vi "Experiment RT Servo.vi"(10 "Experiment Inputs":T2={"Duration"=5.0, "Initialisation Time"=1.0, "Sample Rate (Hz)"=200.0, "signal_type"=enum."Square", "Frequency"=0.5, "Amplitude"=1.0, "Offset"=2.5, "Velocity_feedback_gain"=0.1, "Feedforward_gain"=0.8, "LED_GAIN"=0.0, "LED_OFFSET"=0.0, "initial_condition"=0.0}) -> (0 "Error Out":errorcluster)   [LabVIEW 2016]
uses:
  Controls/Experiment Inputs.ctl
  Controls/Signal Type.ctl
  RT - Controls/Experiment RT State.ctl
  RT - Controls/Machine Data - RT.ctl
  <vilib>/Platform/TimedLoop/XDataNode/timing_clust.ctl
  <vilib>/Platform/TimedLoop/XDataNode/nitl_modes.ctl
  <vilib>/Platform/TimedLoop/XDataNode/wakeup.ctl
  Controller/Controller Values.ctl
  Controls/Experiment Outputs.ctl
  Pauseable Timer/Timer Mode.ctl
  <vilib>/Platform/TimedLoop/XDataNode/XDataNode.xnode
  <vilib>/ptbypt/NI_PtbyPt.lvlib
  <vilib>/Platform/TimedLoop/XDataNode/XDNodeRunTimeDep.lvlib
panel:
  out "Experiment RT State":T1
  in  "Error In":errorcluster
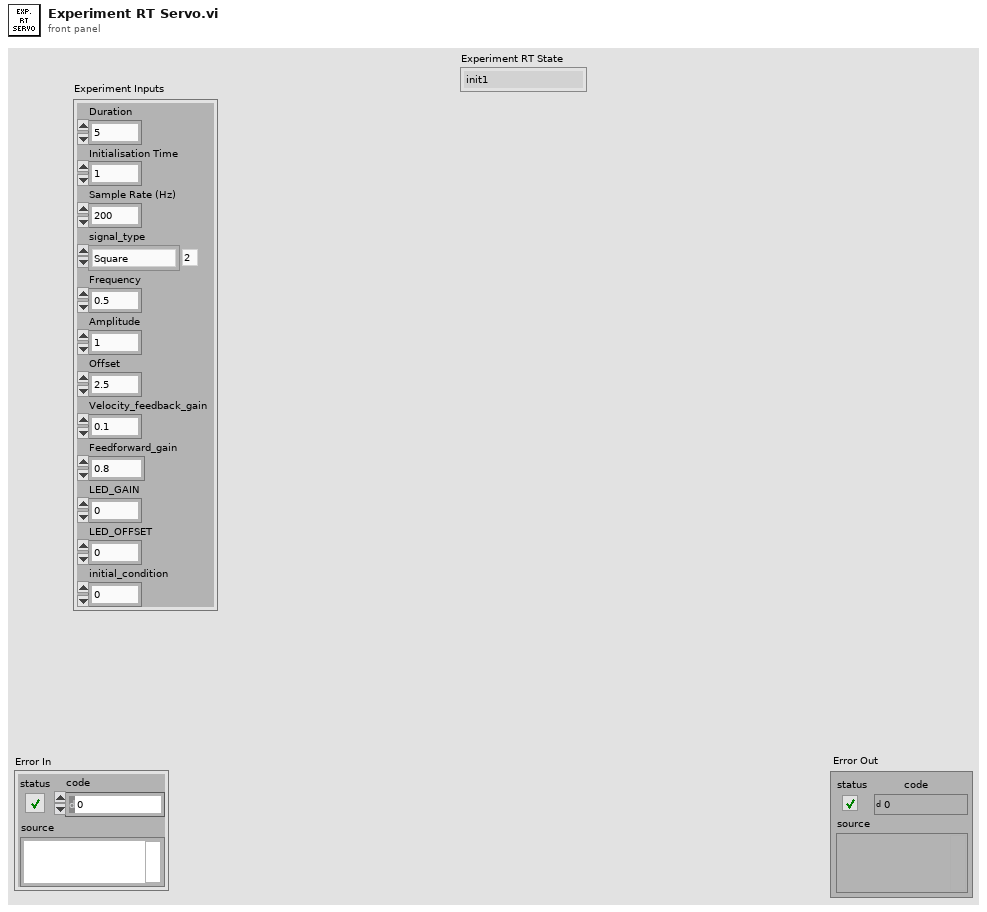
[diagram p1: front panel]
types:
  T1 = typedef "Experiment RT State.ctl" = enum16{"init1", "wait", "setup", "Initialise", "Wait Initialise", "Experiment", "End Experiment", "publisharray1", "publisharray2", "publisharray3", "publishspreadsheet"}
  T2 = typedef "Experiment Inputs.ctl" = cluster{"Duration":dbl, "Initialisation Time":dbl, "Sample Rate (Hz)":dbl, "signal_type":T3, "Frequency":dbl, "Amplitude":dbl, "Offset":dbl, "Velocity_feedback_gain":dbl, "Feedforward_gain":dbl, "LED_GAIN":dbl, "LED_OFFSET":dbl, "initial_condition":dbl}
  T3 = typedef "Signal Type.ctl" = enum16{"Sine", "Cosine", "Square", "Step"}
  T4 = typedef "Machine Data - RT.ctl" = cluster{"Results Array":dbl[][], "Motor Output":dbl, "LED Output":dbl, "Sample Index":u32, "Req. Samples":u32}
  T5 = typedef "XDNodeRunTimeDep.lvlib/timing_clust.ctl" = cluster{"Expected End [f-1]":u64, "Actual End [f-1]":u64, "Finished Late? [f-1]":bool, "Expected End [i-1]":u64, "Actual End [i-1]":u64, "Finished Late? [i-1]":bool, "Expected Start [i]":u64, "Actual Start [i]":u64, "Expected Start [f]":u64, "Actual Start [f]":u64, "Source Name":string, "Structure Name":string, "Period":i64, "Deadline":i64, "Offset":i64, "Start":i64, "Priority":i32, "Timeout":i32, "Mode":T6, "Wakeup Reason":T7, "Error":errorcluster, "Source Type":string, "Secondary Source Type":string, "Global End Time":u64, "Global Start Time":u64, "Frame Duration":u64, "Iteration Duration":u64, "Assigned CPU":i32, "I/O Scan Engine Mode":u32}
  T6 = typedef "XDNodeRunTimeDep.lvlib/nitl_modes.ctl" = enum32{"No Change", "Process missed periods, maintain original phase", "Discard missed periods, maintain original phase", "Process missed periods, ignore original phase", "Discard missed periods, ignore original phase"}
  T7 = typedef "XDNodeRunTimeDep.lvlib/wakeup.ctl" = enum32{"Normal", "Aborted", "Asynchronous wakeup", "Timing source error", "Timed loop error", "Timeout"}
  T8 = typedef "Controller Values.ctl" = cluster{"Ka":dbl, "Kt":dbl, "Offset":dbl}
  T9 = typedef "Timer Mode.ctl" = enum16{"Initialise", "Read", "Pause"}
  T10 = typedef "Experiment Outputs.ctl" = cluster{"Results Array":dbl[][], "spreadsheet":string}
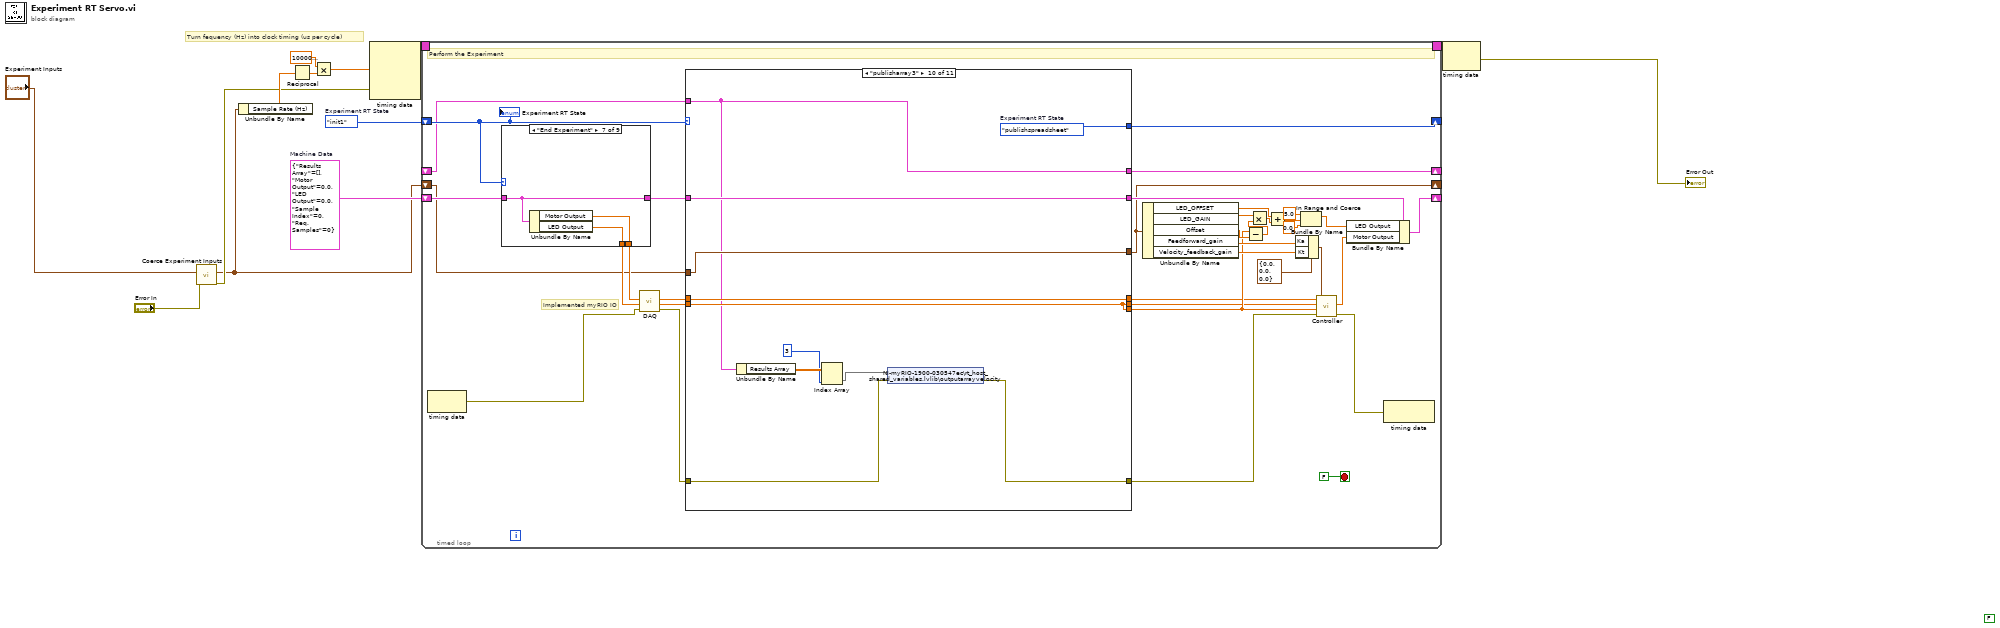
[diagram p0: block diagram]
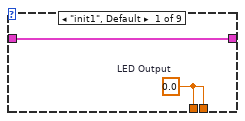
[diagram p2: hidden frame]
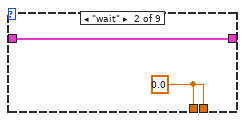
[diagram p3: hidden frame]
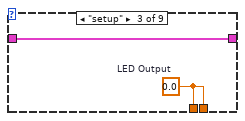
[diagram p4: hidden frame]
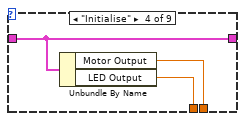
[diagram p5: hidden frame]
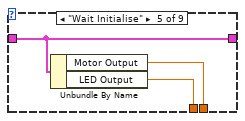
[diagram p6: hidden frame]
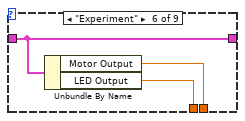
[diagram p7: hidden frame]
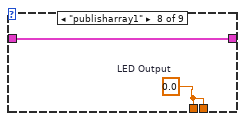
[diagram p8: hidden frame]
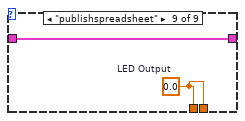
[diagram p9: hidden frame]
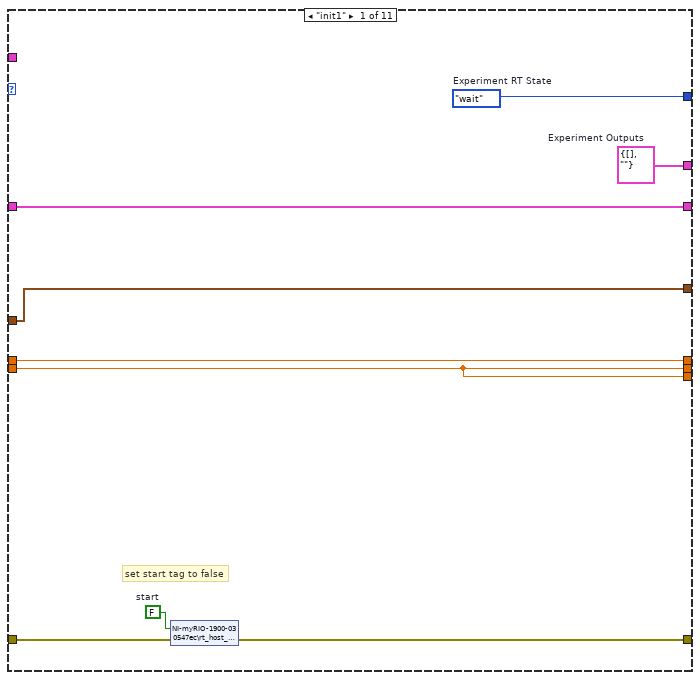
[diagram p10: hidden frame]
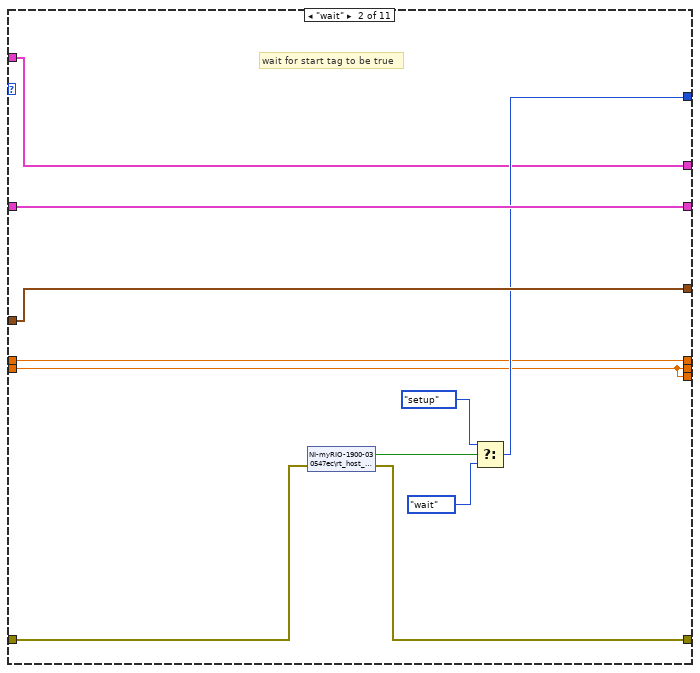
[diagram p11: hidden frame]
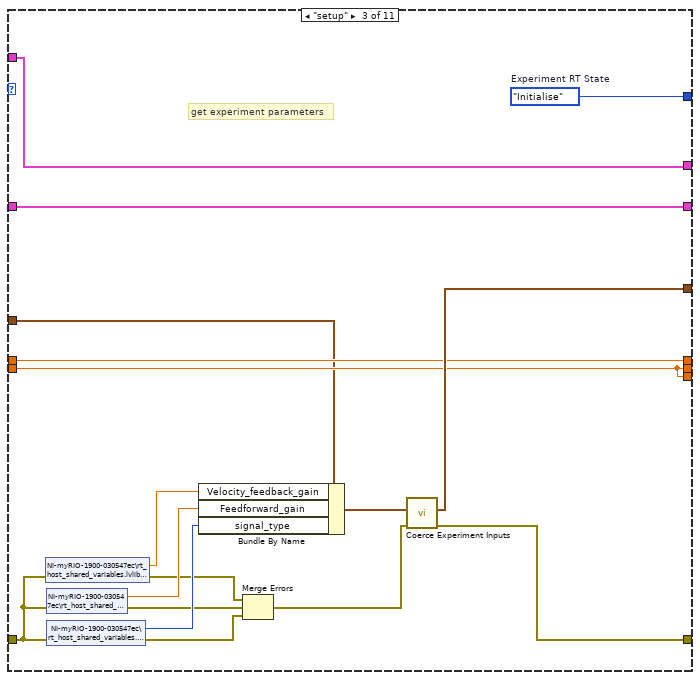
[diagram p12: hidden frame]
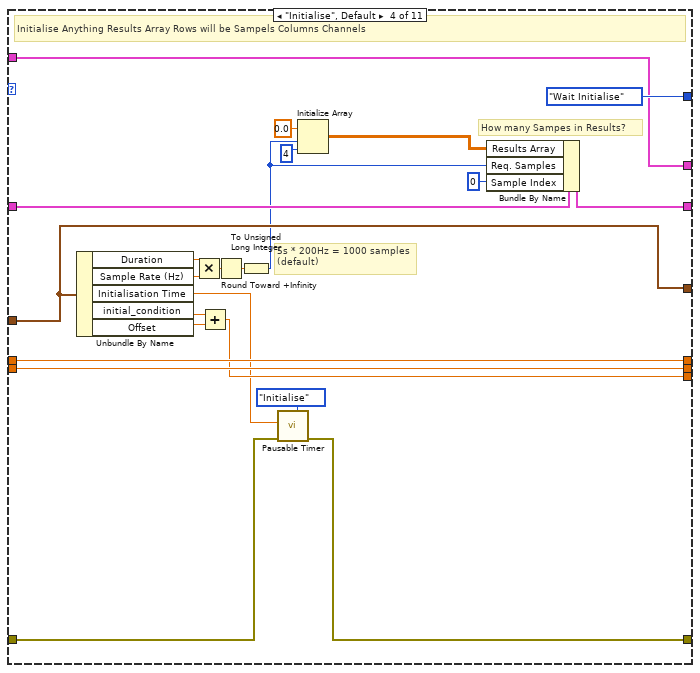
[diagram p13: hidden frame]
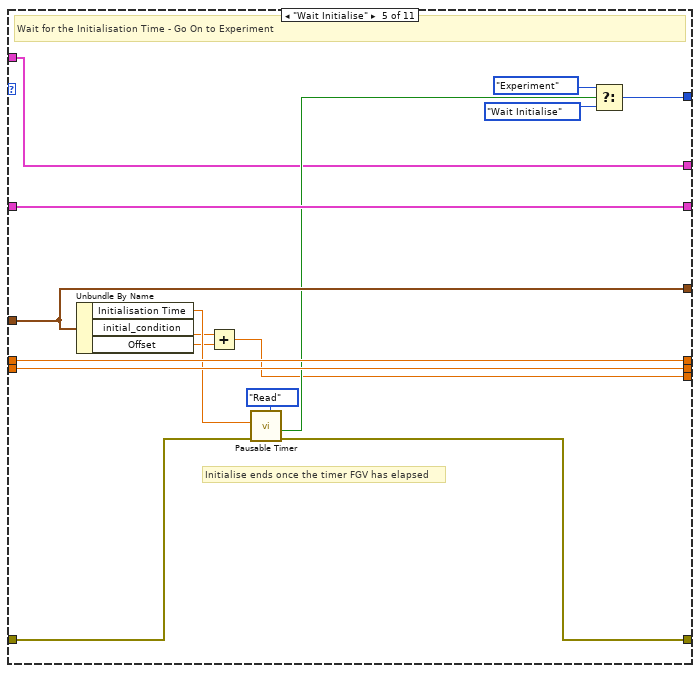
[diagram p14: hidden frame]
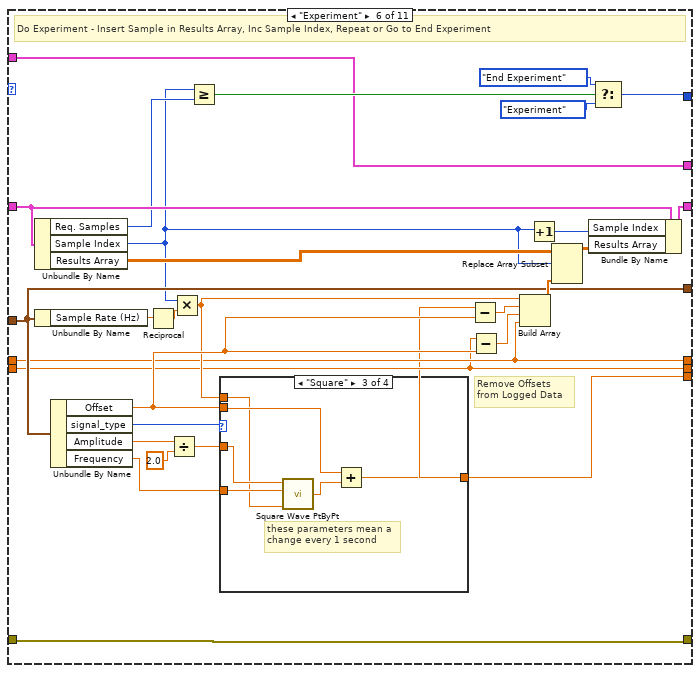
[diagram p15: hidden frame]
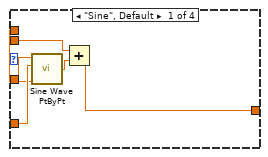
[diagram p16: hidden frame]
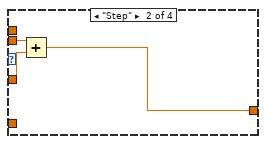
[diagram p17: hidden frame]
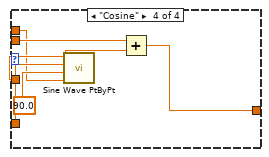
[diagram p18: hidden frame]
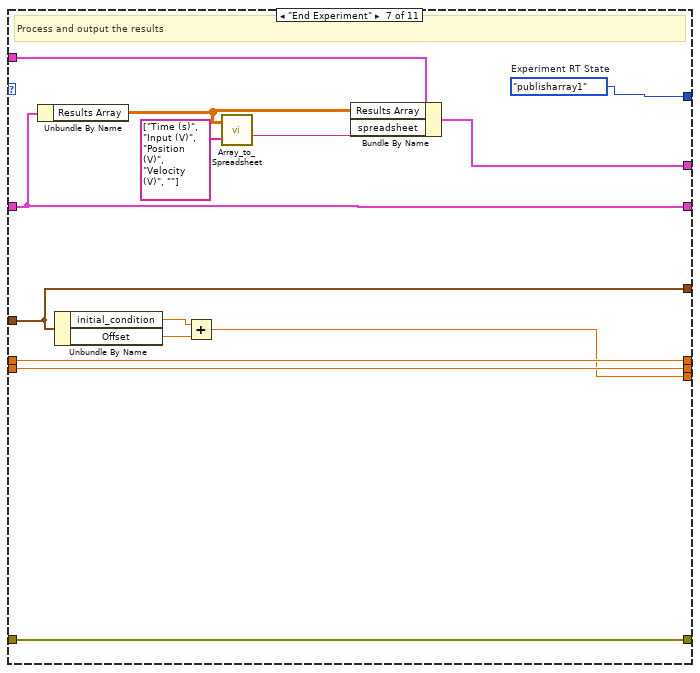
[diagram p19: hidden frame]
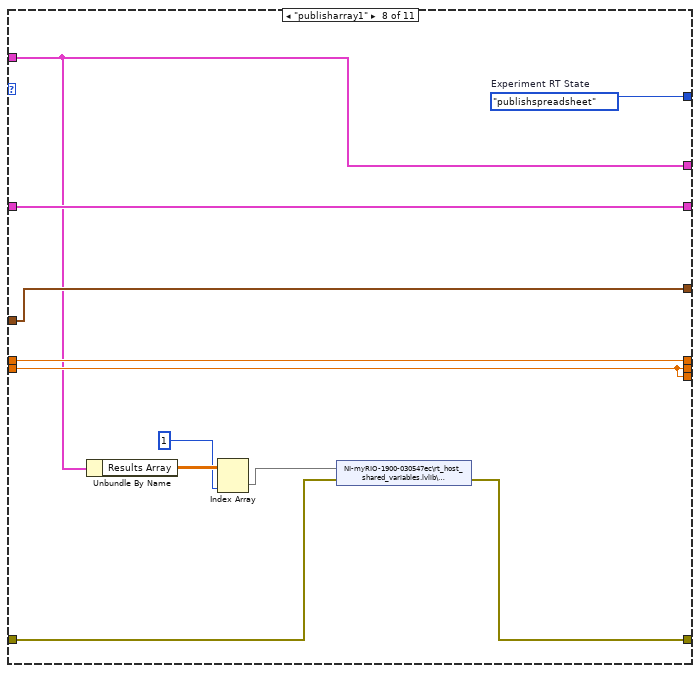
[diagram p20: hidden frame]
diagram:
  (unwired) FALSE
  w5 = T4 {"Results Array"=[], "Motor Output"=0.0, "LED Output"=0.0, "Sample Index"=0, "Req. Samples"=0}  # Machine Data
  w11 = Experiment_RT_State."init1"  # Experiment RT State
  # "Turn fequency (Hz) into clock timing (us per cycle)"
  n1 = call "Coerce Experiment Inputs.vi"("Error In"="Error In", "Experiment Inputs"="Experiment Inputs") -> ("Error Out"=w6:errorcluster, "Experiment Inputs Out"=w1:T2)  [unwired: 8 in]
  n2 = Unbundle By Name(w1) -> ("Sample Rate (Hz)"=w10:dbl)
  n3 = Reciprocal(x=w10) -> (1/x=w9:dbl)
  n4 = Multiply(x=1000000.0 ("y"), y=w9) -> (x*y=w7:dbl)
  n5 = node-c288(w7, w6) -> (w13:T5)  [unwired: 2 in]
  n6 = timed-loop {
    shift-right: [w45] -> _
    shift-left: w11 -> [w17]
    shift-right: [w48] -> _
    shift-left: w5 -> [w49]
    timing: w13 -> [_]
    timing-out: [_] -> w12
    shift-right: [w32] -> _
    shift-left: w1 -> [w18]
    shift-right: [w44] -> _
    shift-left: _ -> [w15]
    stop <- FALSE stop-if-true
    # "Implemented myRIO IO"
    # "Perform the Experiment"
    n7 = node-c288() -> (w46:errorcluster)  [unwired: 1 in]
    n8 = case shown="\"End Experiment\"" w17 {
      tunnel: w49 -> [w51 w53 w55 w58 w61 w64 w67 w69 w71]
      tunnel: [w50 w52 w54 w57 w60 w63 w66 w68 w70] -> w36
      tunnel: [w50 w52 w54 w56 w59 w62 w65 w68 w70] -> w22
      tunnel: [w51 w53 w55 w58 w61 w64 w67 w69 w71] -> w16
      frame "init1", Default {
        w50 = 0.0  # LED Output
      }
      frame "wait" {
        w52 = 0.0
      }
      frame "setup" {
        w54 = 0.0  # LED Output
      }
      frame "Initialise" {
        n9 = Unbundle By Name(w58) -> ("Motor Output"=w56:dbl, "LED Output"=w57:dbl)
      }
      frame "Wait Initialise" {
        n10 = Unbundle By Name(w61) -> ("Motor Output"=w59:dbl, "LED Output"=w60:dbl)
      }
      frame "Experiment" {
        n11 = Unbundle By Name(w64) -> ("Motor Output"=w62:dbl, "LED Output"=w63:dbl)
      }
      frame "End Experiment" {
        n12 = Unbundle By Name(w67) -> ("Motor Output"=w65:dbl, "LED Output"=w66:dbl)
      }
      frame "publisharray1" {
        w68 = 0.0  # LED Output
      }
      frame "publishspreadsheet" {
        w70 = 0.0  # LED Output
      }
    }
    n13 = call "DAQ.vi"("Error In"=w46, "LED Output"=w36, "Motor Output"=w22) -> ("Error Out"=w38:errorcluster, "Position FB"=w23:dbl, "Tacho FB"=w24:dbl)  [unwired: 4 in, 2 out]
    n14 = case shown="\"publisharray3\"" w17 {
      tunnel: [w72 w88 w107 w129 w147 w161 w200 w214 w226 w236 w249] -> w43
      tunnel: w18 -> [w78 w91 w101 w125 w146 w165 w210 w221 w232 w243 w252]
      tunnel: w16 -> [w75 w90 w103 w131 w142 w176 w209 w222 w233 w244 w253]
      tunnel: [w75 w90 w103 w130 w142 w175 w209 w222 w233 w244 w253] -> w37
      tunnel: [w78 w91 w106 w125 w146 w165 w210 w221 w232 w243 w252] -> w32
      tunnel: w38 -> [w79 w89 w102 w123 w145 w161 w200 w213 w225 w235 w250]
      tunnel: [w76 w82 w104 w124 w134 w149 w204 w219 w230 w241 w251] -> w25
      tunnel: w24 -> [w77 w83 w105 w128 w144 w156 w212 w220 w231 w242 w251]
      tunnel: [w77 w83 w105 w128 w144 w156 w212 w220 w231 w242 w251] -> w20
      tunnel: [w76 w82 w104 w127 w143 w155 w211 w219 w230 w241 w251] -> w19
      tunnel: w23 -> [w76 w82 w104 w127 w143 w155 w211 w219 w230 w241 _]
      tunnel: [w73 w84 w108 Experiment_RT_State."Wait Initialise" ("Experiment RT State") w141 w173 w199 w223 w234 w245 w254] -> w45
      tunnel: [w74 w81 w92 w109 w132 w148 w202 w218 w229 w240 w247] -> w44
      tunnel: w15 -> [_ w81 w92 w109 w132 w148 w201 w218 w229 w240 w247]
      frame "init1" {
        w73 = Experiment_RT_State."wait"  # Experiment RT State
        w74 = T10 {"Results Array"=[], "spreadsheet"=""}  # Experiment Outputs
        w80 = FALSE  # start
        # "set start tag to false"
        n15 = shared-variable "NI-myRIO-1900-030547ec\\rt_host_shared_variables.lvlib\\start"(w80, error in=w79) -> (error out=w72:errorcluster)
      }
      frame "wait" {
        # "wait for start tag to be true"
        n16 = shared-variable "NI-myRIO-1900-030547ec\\rt_host_shared_variables.lvlib\\start"(error in=w89) -> (w87:bool, error out=w88:errorcluster)
        n17 = Select(t=Experiment_RT_State."setup" ("Experiment RT State"), s=w87, f=Experiment_RT_State."wait" ("Experiment RT State")) -> (s? t:f=w84:T1)
      }
      frame "setup" {
        w108 = Experiment_RT_State."Initialise"  # Experiment RT State
        # "get experiment parameters"
        n18 = shared-variable "NI-myRIO-1900-030547ec\\rt_host_shared_variables.lvlib\\vel_fb_gain"(error in=w102) -> (w100:dbl, error out=w96:errorcluster)
        n19 = shared-variable "NI-myRIO-1900-030547ec\\rt_host_shared_variables.lvlib\\ff_gain"(error in=w102) -> (w99:dbl, error out=w95:errorcluster)
        n20 = shared-variable "NI-myRIO-1900-030547ec\\rt_host_shared_variables.lvlib\\signaltype"(error in=w102) -> (w98:u32, error out=w94:errorcluster)
        n21 = Bundle By Name(cluster=w101, "Velocity_feedback_gain"=w100, "Feedforward_gain"=w99, "signal_type"=w98) -> (w97:T2)
        n22 = Merge Errors(w96, w95, w94) -> (w93:errorcluster)
        n23 = call "Coerce Experiment Inputs.vi"("Error In"=w93, "Experiment Inputs"=w97) -> ("Error Out"=w107:errorcluster, "Experiment Inputs Out"=w106:T2)  [unwired: 8 in]
      }
      frame "Initialise", Default {
        # "5s * 200Hz = 1000 samples\n(default)"
        # "How many Sampes in Results?"
        # "Initialise Anything Results Array Rows will be Sampels Columns Channels"
        n24 = Unbundle By Name(w125) -> ("Duration"=w121:dbl, "Sample Rate (Hz)"=w120:dbl, "Initialisation Time"=w122:dbl, "initial_condition"=w112:dbl, "Offset"=w111:dbl)
        n25 = Multiply(x=w121, y=w120) -> (x*y=w119:dbl)
        n26 = Add(x=w112, y=w111) -> (x+y=w124:dbl)
        n27 = Round Toward +Infinity(x=w119) -> (ceil(x): smallest int >= x=w118:dbl)
        n28 = To Unsigned Long Integer(number=w118) -> (unsigned 32bit integer=w113:u32)
        n29 = call "Pausable Timer.vi"("Timer Mode"=Timer_Mode."Initialise", "Error In"=w123, "Desired Time (S)"=w122) -> ("Error Out"=w129:errorcluster)  [unwired: 6 in, 2 out]
        n30 = Initialize Array(0.0 ("element"), w113, 4 ("dimension size")) -> (w115:dbl[][])
        n31 = Bundle By Name(cluster=w131, "Results Array"=w115, "Req. Samples"=w113, "Sample Index"=u32 0) -> (w130:T4)
      }
      frame "Wait Initialise" {
        # "Initialise ends once the timer FGV has elapsed"
        # "Wait for the Initialisation Time - Go On to Experiment"
        n32 = Unbundle By Name(w146) -> ("Initialisation Time"=w140:dbl, "initial_condition"=w135:dbl, "Offset"=w133:dbl)
        n33 = Add(x=w135, y=w133) -> (x+y=w134:dbl)
        n34 = call "Pausable Timer.vi"("Timer Mode"=Timer_Mode."Read", "Error In"=w145, "Desired Time (S)"=w140) -> ("Error Out"=w147:errorcluster, "Time Up?"=w139:bool)  [unwired: 6 in, 1 out]
        n35 = Select(t=Experiment_RT_State."Experiment" ("Experiment RT State"), s=w139, f=Experiment_RT_State."Wait Initialise" ("Experiment RT State")) -> (s? t:f=w141:T1)
      }
      frame "Experiment" {
        # "Remove Offsets\nfrom Logged Data"
        # "Do Experiment - Insert Sample in Results Array, Inc Sample Index, Repeat or Go to End Experiment"
        n36 = Unbundle By Name(w176) -> ("Req. Samples"=w169:u32, "Sample Index"=w164:u32, "Results Array"=w167:dbl[][])
        n37 = Unbundle By Name(w165) -> ("Sample Rate (Hz)"=w163:dbl)
        n38 = Unbundle By Name(w165) -> ("Offset"=w158:dbl, "signal_type"=w160:T3, "Amplitude"=w151:dbl, "Frequency"=w159:dbl)
        n39 = Reciprocal(x=w163) -> (1/x=w162:dbl)
        n40 = Divide(x=w151, y=2.0) -> (x/y=w152:dbl)
        n41 = Multiply(x=w164, y=w162) -> (x*y=w157:dbl)
        n42 = Greater Or Equal?(x=w164, y=w169) -> (x >= y?=w170:bool)
        n43 = case shown="\"Square\"" w160 {
          tunnel: w152 -> [w182 w184 w191 w197]
          tunnel: w159 -> [w181 _ w190 w196]
          tunnel: w158 -> [w179 w185 w188 w193]
          tunnel: [w178 w183 w186 w194] -> w149
          tunnel: w157 -> [w177 _ w187 w192]
          frame "Sine", Default {
            n44 = call <vilib>:"Sine Wave PtByPt.vi"("time"=w177, "frequency"=w181, "amplitude"=w182) -> ("sine wave"=w180:dbl)  [unwired: 1 in]
            n45 = Add(x=w179, y=w180) -> (x+y=w178:dbl)
          }
          frame "Step" {
            n46 = Add(x=w185, y=w184) -> (x+y=w183:dbl)
          }
          frame "Square" {
            # "these parameters mean a\nchange every 1 second"
            n47 = call <vilib>:"Square Wave PtByPt.vi"("amplitude"=w191, "frequency"=w190, "time"=w187) -> ("square wave"=w189:dbl)  [unwired: 2 in]
            n48 = Add(x=w188, y=w189) -> (x+y=w186:dbl)
          }
          frame "Cosine" {
            n49 = call <vilib>:"Sine Wave PtByPt.vi"("time"=w192, "phase"=90.0, "frequency"=w196, "amplitude"=w197) -> ("sine wave"=w195:dbl)
            n50 = Add(x=w193, y=w195) -> (x+y=w194:dbl)
          }
        }
        n51 = Subtract(x=w149, y=w158) -> (x-y=w154:dbl)
        n52 = Subtract(x=w155, y=w158) -> (x-y=w153:dbl)
        n53 = Build Array(w157, w154, w153, w156) -> (w166:dbl[])
        n54 = Increment(x=w164) -> (x+1=w174:u32)
        n55 = Replace Array Subset(array=w167, new element=w166, index (row)=w164) -> (w168:dbl[][])  [unwired: 1 in]
        n56 = Bundle By Name(cluster=w176, "Sample Index"=w174, "Results Array"=w168) -> (w175:T4)
        n57 = Select(t=Experiment_RT_State."End Experiment" ("Experiment RT State"), s=w170, f=Experiment_RT_State."Experiment" ("Experiment RT State")) -> (s? t:f=w173:T1)
      }
      frame "End Experiment" {
        w199 = Experiment_RT_State."publisharray1"  # Experiment RT State
        # "Process and output the results"
        n58 = Unbundle By Name(w209) -> ("Results Array"=w203:dbl[][])
        n59 = Unbundle By Name(w210) -> ("initial_condition"=w205:dbl, "Offset"=w206:dbl)
        n60 = Add(x=w205, y=w206) -> (x+y=w204:dbl)
        n61 = call "Array_to_Spreadsheet.vi"("Headers"=string[] ["Time (s)", "Input (V)", "Position (V)", "Velocity (V)", ""], "Input Array"=w203) -> ("spreadsheet string"=w208:string)
        n62 = Bundle By Name(cluster=w201, "Results Array"=w203, "spreadsheet"=w208) -> (w202:T10)
      }
      frame "publisharray1" {
        w223 = Experiment_RT_State."publishspreadsheet"  # Experiment RT State
        n63 = Unbundle By Name(w218) -> ("Results Array"=w217:dbl[][])
        n64 = Index Array(array=w217, index (col)=1 ("disabled index (col)")) -> (element=w215:dbl[])  [unwired: 1 in]
        n65 = shared-variable "NI-myRIO-1900-030547ec\\rt_host_shared_variables.lvlib\\outputarrayinput"(w215, error in=w213) -> (error out=w214:errorcluster)
      }
      frame "publisharray2" {
        w234 = Experiment_RT_State."publishspreadsheet"  # Experiment RT State
        n66 = Unbundle By Name(w229) -> ("Results Array"=w228:dbl[][])
        n67 = Index Array(array=w228, index (col)=2 ("disabled index (col)")) -> (element=w224:dbl[])  [unwired: 1 in]
        n68 = shared-variable "NI-myRIO-1900-030547ec\\rt_host_shared_variables.lvlib\\outputarrayposition"(w224, error in=w225) -> (error out=w226:errorcluster)
      }
      frame "publisharray3" {
        w245 = Experiment_RT_State."publishspreadsheet"  # Experiment RT State
        n69 = Unbundle By Name(w240) -> ("Results Array"=w239:dbl[][])
        n70 = Index Array(array=w239, index (col)=3 ("disabled index (col)")) -> (element=w237:dbl[])  [unwired: 1 in]
        n71 = shared-variable "NI-myRIO-1900-030547ec\\rt_host_shared_variables.lvlib\\outputarrayvelocity"(w237, error in=w235) -> (error out=w236:errorcluster)
      }
      frame "publishspreadsheet" {
        w254 = Experiment_RT_State."init1"  # Experiment RT State
        n72 = Unbundle By Name(w247) -> ("spreadsheet"=w246:string)
        n73 = To Variant(anything=w246) -> (Variant=w248:variant)
        n74 = shared-variable "NI-myRIO-1900-030547ec\\rt_host_shared_variables.lvlib\\Output"(w248, error in=w250) -> (error out=w249:errorcluster)
      }
    }
    n75 = Unbundle By Name(w32) -> ("LED_OFFSET"=w33:dbl, "LED_GAIN"=w35:dbl, "Offset"=w30:dbl, "Feedforward_gain"=w40:dbl, "Velocity_feedback_gain"=w39:dbl)
    n76 = Subtract(x=w25, y=w30) -> (x-y=w31:dbl)
    n77 = Multiply(x=w35, y=w31) -> (x*y=w34:dbl)
    n78 = Add(x=w33, y=w34) -> (x+y=w29:dbl)
    n79 = Bundle By Name(cluster=T8 {"Ka"=0.0, "Kt"=0.0, "Offset"=0.0} ("Controller Values"), "Ka"=w40, "Kt"=w39) -> (w41:T8)
    n80 = In Range and Coerce(upper limit=5.0, x=w29, lower limit=0.0) -> (coerced(x)=w26:dbl)  [unwired: 1 out]
    n81 = call "Controller.vi"("Controller Values"=w41, "Error In"=w43, "Set Point"=w25, "Position FB"=w19, "Tacho FB"=w20) -> ("Error Out"=w47:errorcluster, "Controller Out"=w21:dbl)  [unwired: 5 in]
    n82 = Bundle By Name(cluster=w37, "LED Output"=w26, "Motor Output"=w21) -> (w48:T4)
    n83 = node-c288(w47) -> ()  [unwired: 1 out]
    "Experiment RT State" <- w17
  }
  n84 = node-c288(w12) -> (→"Error Out":errorcluster)
